vi "FSRCalibrationDataCollection.vi"() -> ()   [LabVIEW 2020]
doc: "Use this template to build a producer/consumer design pattern. Use this template when you need to execute a process, such as data analysis, when a data source, such as a triggered acquisition, produces data at an uneven rate and you need to execute the process when the data becomes available.\n------------------------------------\nAuther: Koji Ohashi\nCopyright (c) 2020 Japan LabVIEW Users Group, Volunteer members.\nThis VI is released under the MIT License.\nhttp://opensource.org/licenses/mit-license.php\n------------------------------------"
uses:
  FSRCalibrationDataCollection Folder/For fsr type def.ctl
  <vilib>/Analysis/baseanly.llb/Mean (DBL).vi
  <vilib>/Instr/_visa.llb/VISA Configure Serial Port (Instr).vi
  <vilib>/Analysis/NI_AALBase.lvlib
panel:
  out "Vout F4":dbl(slide) scale=0.0..2000.0
  out "Collecting":bool
  in  "Timer [ms]":u32
  out "On Time [ms]":u32
  out "millisecond timer":u32
  in  "Weight":T1(ring)
  out "Vout F1":dbl(slide) scale=0.0..2000.0
  in  "?":bool
  in  "Weight":string
  in  "Path":path=path "C:/Users/rsKite/Documents/FSR DATA"
  in  "Trial":string caption="Participant Name (FirstLast)"
  out "File Name":string
  out "Vout F3":dbl(slide) scale=0.0..2000.0
  out "Vout F2":dbl(slide) scale=0.0..2000.0
  out "Status":string
  in  "?":bool
  in  "VISA resource name":refnum<visa-resource-name>="COM1"
  in  "stop":bool
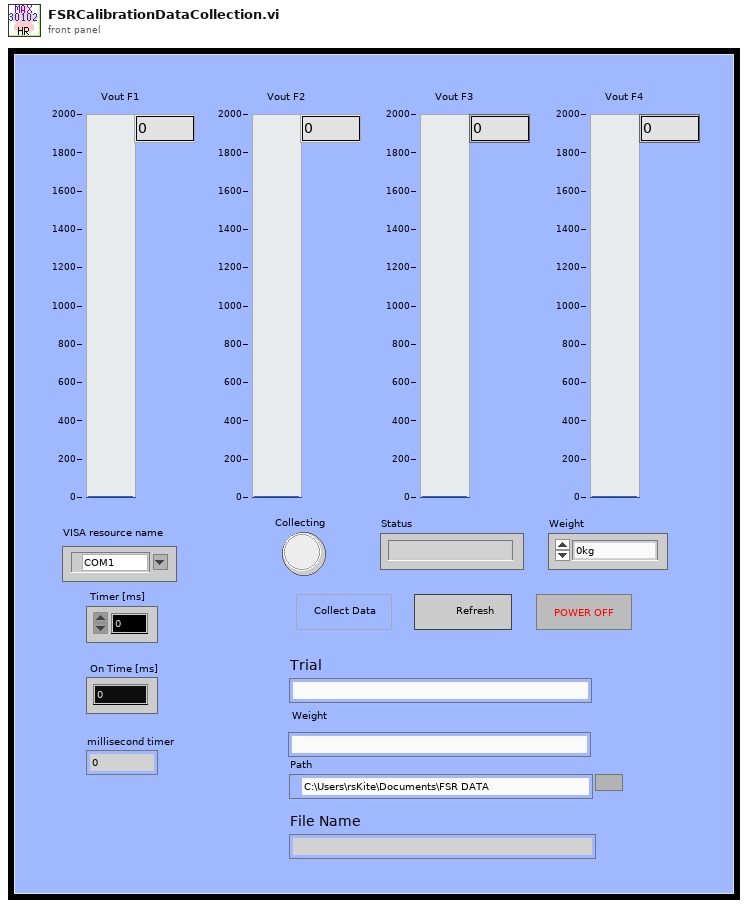
[diagram p1: front panel]
types:
  T1 = enum16{"0kg", "0.1kg", "0.2kg", "0.3kg", "0.4kg", "0.5kg", "0.6kg", "0.7kg", "0.8kg", "0.9kg", "1kg", "1.1kg", "1.2kg", "1.3kg", "1.4kg", "1.5kg", "1.6kg", "1.7kg", "1.8kg", "1.9kg", "2.0kg"}
  T2 = enum16{"open", "replace", "create", "open or create", "replace or create", "replace or create with confirmation"}
  T3 = typedef "For fsr type def.ctl" = enum16{"Create/Replace File", "Waiting Room", "Collect Data", "Write Data", "Close File", "Reinit"}
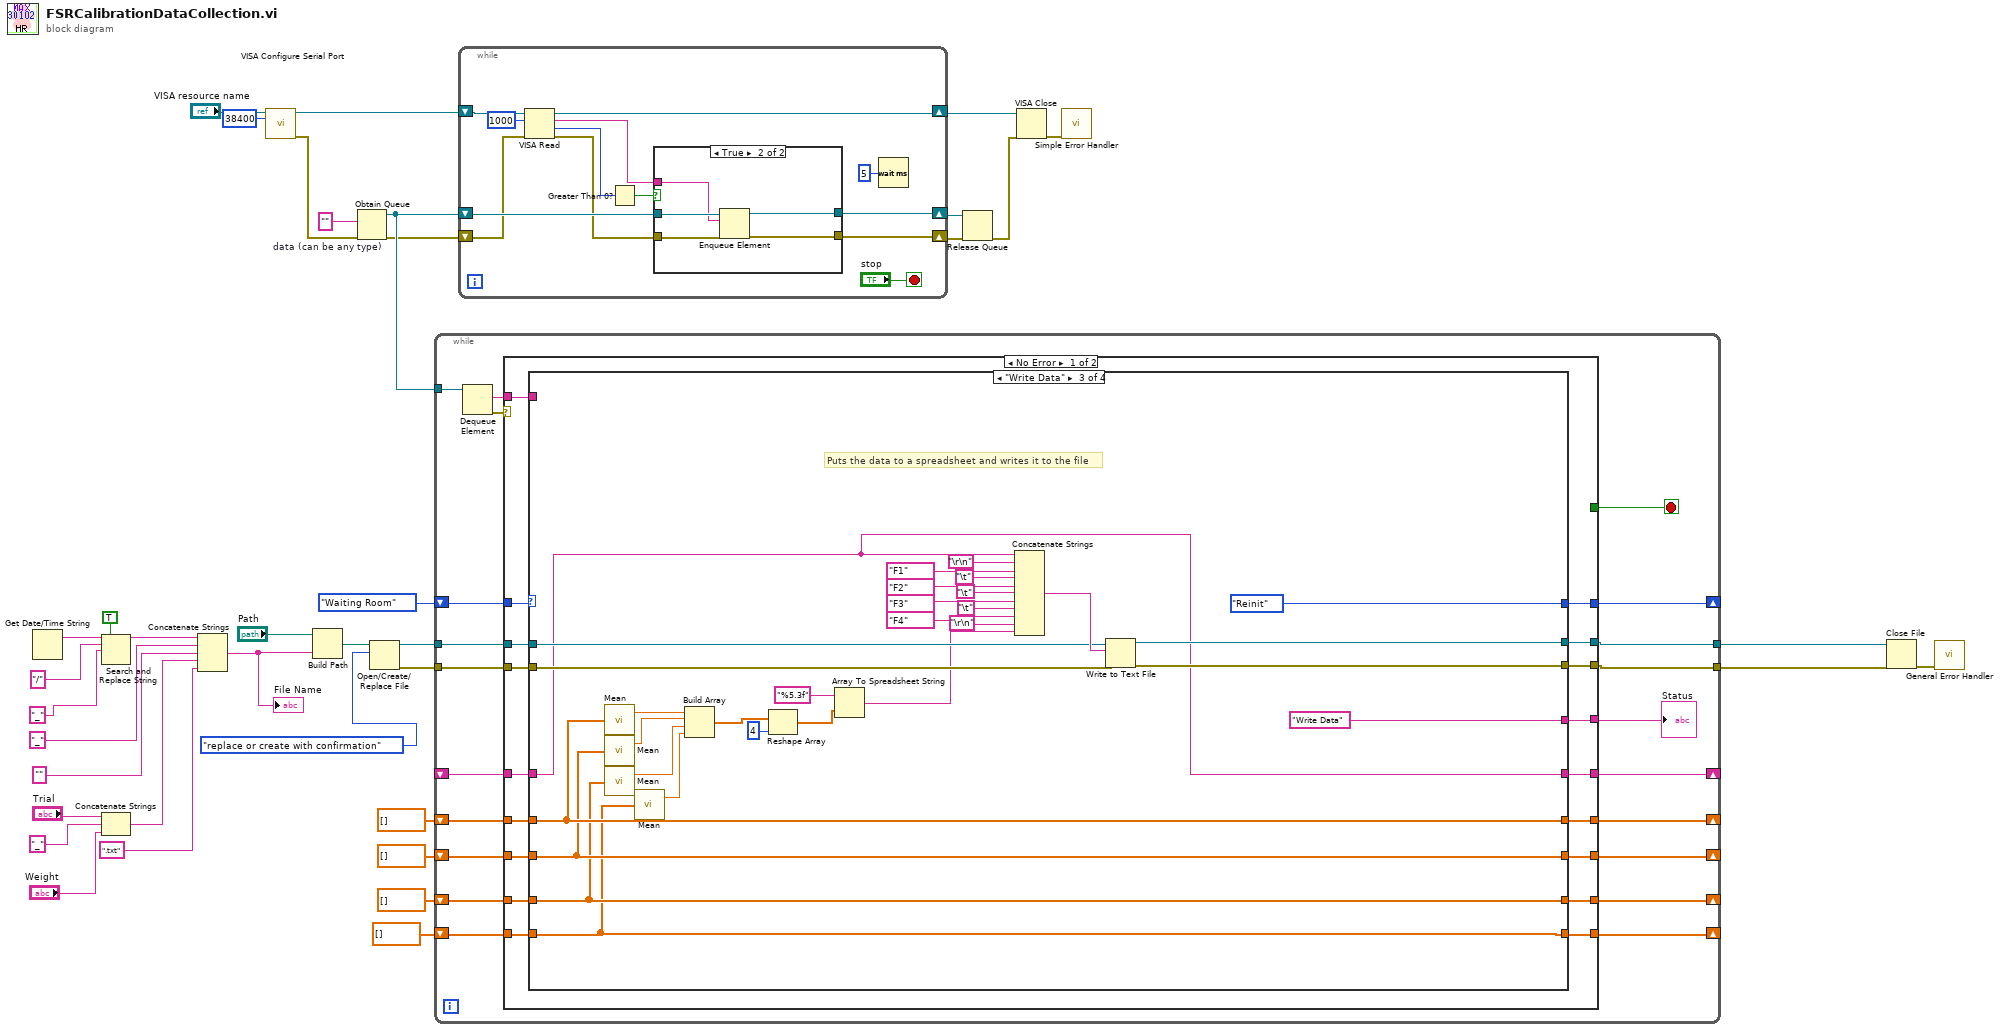
[diagram p0: block diagram]
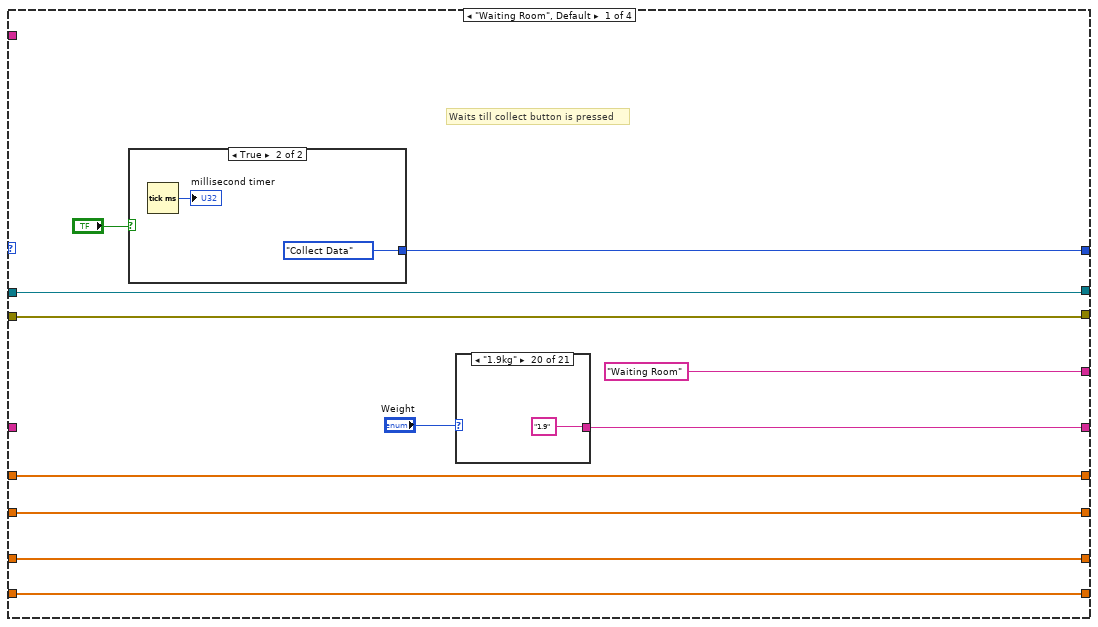
[diagram p2: hidden frame]
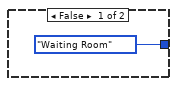
[diagram p3: hidden frame]
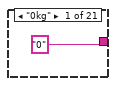
[diagram p4: hidden frame]
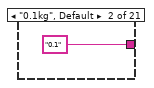
[diagram p5: hidden frame]
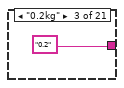
[diagram p6: hidden frame]
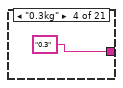
[diagram p7: hidden frame]
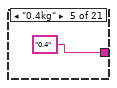
[diagram p8: hidden frame]
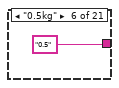
[diagram p9: hidden frame]
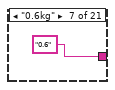
[diagram p10: hidden frame]
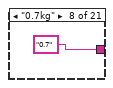
[diagram p11: hidden frame]
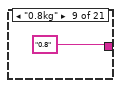
[diagram p12: hidden frame]
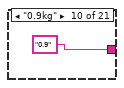
[diagram p13: hidden frame]
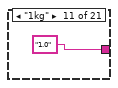
[diagram p14: hidden frame]
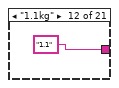
[diagram p15: hidden frame]
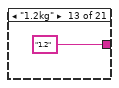
[diagram p16: hidden frame]
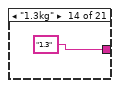
[diagram p17: hidden frame]
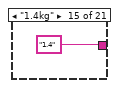
[diagram p18: hidden frame]
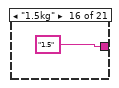
[diagram p19: hidden frame]
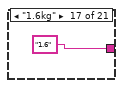
[diagram p20: hidden frame]
diagram:
  w34 = ""  # data (can be any type)
  n1 = Get Date/Time String() -> (date string=w25:string)  [unwired: 3 in, 1 out]
  n2 = Search and Replace String(replace all?=TRUE ("replace all? (F)"), input string=w25, search string="/", replace string="_" ("replace string (\"\")")) -> (result string=w23:string)  [unwired: 4 in, 3 out]
  n3 = Concatenate Strings("Trial", "_" ("string"), "Weight") -> (w24:string)
  n4 = Concatenate Strings(w23, "_" ("string"), "" ("string"), w24, ".txt" ("string")) -> (w21:string)
  "File Name" <- w21
  n5 = call-poly "VISA Configure Serial Port"("VISA resource name"="VISA resource name", "baud rate (9600)"=u32 38400) -> ("VISA resource name out"=w32:refnum<visa-resource-name>, "error out"=w29:errorcluster)  [unwired: 8 in, 4 out]
  n6 = Build Path(base path="Path", name or relative path=w21) -> (appended path=w10:path)
  n7 = Obtain Queue(element data type=w34, error in (no error)=w29) -> (queue out=w38:refnum<queue>, error out=w37:errorcluster)  [unwired: 3 in, 1 out]
  n8 = Open/Create/Replace File(file path (use dialog)=w10, operation (0:open)=T2."replace or create with confirmation") -> (refnum out=w8:refnum<file>, error out=w7:errorcluster)  [unwired: 4 in, 1 out]
  n9 = while {
    tunnel: w38 -> [w59]
    shift-right: [w53] -> _
    shift-left: For_fsr_type_def."Waiting Room" -> [w54]
    tunnel: w8 -> [w52]
    tunnel: w7 -> [w51]
    tunnel: [w50] -> w6
    tunnel: [w49] -> w5
    shift-right: [w45] -> _
    shift-left: dbl[] [] -> [w46]
    shift-right: [w47] -> _
    shift-left: dbl[] [] -> [w48]
    shift-right: [w43] -> _
    shift-left: dbl[] [] -> [w44]
    shift-right: [w41] -> _
    shift-left: _ -> [w42]
    shift-right: [w39] -> _
    shift-left: dbl[] [] -> [w40]
    stop <- w56 stop-if-true
    n10 = Dequeue Element(queue=w59) -> (element=w57:string, error out=w58:errorcluster)  [unwired: 2 in, 2 out]
    n11 = case shown="No Error" w58 {
      tunnel: w57 -> [w75 _]
      tunnel: [_ TRUE] -> w56
      tunnel: [w74 "Error or POWER OFF"] -> w55
      tunnel: w54 -> [w77 _]
      tunnel: [w76 For_fsr_type_def."Waiting Room"] -> w53
      tunnel: w52 -> [w73 w211]
      tunnel: w51 -> [w72 w210]
      tunnel: [w71 w211] -> w50
      tunnel: [w70 w210] -> w49
      tunnel: w48 -> [w69 w207]
      tunnel: [w68 w207] -> w47
      tunnel: w46 -> [w67 w208]
      tunnel: [w66 w208] -> w45
      tunnel: w44 -> [w65 w209]
      tunnel: [w64 w209] -> w43
      tunnel: w42 -> [w63 w206]
      tunnel: [w62 w206] -> w41
      tunnel: w40 -> [w61 w205]
      tunnel: [w60 w205] -> w39
      frame No Error {
        n12 = case shown="\"Write Data\"" w77 {
          tunnel: [w80 w122 For_fsr_type_def."Reinit" w189] -> w76
          tunnel: w75 -> [_ w142 _ _]
          tunnel: ["Waiting Room" "Collect data" "Write Data" "Reinit"] -> w74
          tunnel: w73 -> [w87 w140 w169 w191]
          tunnel: w72 -> [w86 w139 w168 w190]
          tunnel: [w87 w140 w167 w191] -> w71
          tunnel: [w86 w139 w166 w190] -> w70
          tunnel: w69 -> [w83 w136 w162 w183]
          tunnel: [w83 w118 w162 w186] -> w68
          tunnel: w67 -> [w84 w133 w163 w184]
          tunnel: [w84 w131 w163 w187] -> w66
          tunnel: w65 -> [w85 w132 w164 w185]
          tunnel: [w85 w130 w164 w188] -> w64
          tunnel: [w82 w128 w154 w180] -> w62
          tunnel: w63 -> [_ w128 w154 w181]
          tunnel: w61 -> [w78 w116 w153 w179]
          tunnel: [w78 w115 w153 w178] -> w60
          frame "Waiting Room", Default {
            # "Waits till collect button is pressed"
            n13 = case shown="True" "?" {
              tunnel: [For_fsr_type_def."Waiting Room" For_fsr_type_def."Collect Data"] -> w80
              frame False {
              }
              frame True {
                n14 = Tick Count (ms)() -> (millisecond timer value=→"millisecond timer":u32)
              }
            }
            n15 = case shown="\"1.9kg\"" "Weight" {
              tunnel: ["0" "0.1" "0.2" "0.3" "0.4" "0.5" "0.6" "0.7" "0.8" "0.9" "1.0" "1.1" "1.2" "1.3" "1.4" "1.5" "1.6" "1.7" "1.8" "1.9" "2.0"] -> w82
              frame "0kg" {
              }
              frame "0.1kg", Default {
              }
              frame "0.2kg" {
              }
              frame "0.3kg" {
              }
              frame "0.4kg" {
              }
              frame "0.5kg" {
              }
              frame "0.6kg" {
              }
              frame "0.7kg" {
              }
              frame "0.8kg" {
              }
              frame "0.9kg" {
              }
              frame "1kg" {
              }
              frame "1.1kg" {
              }
              frame "1.2kg" {
              }
              frame "1.3kg" {
              }
              frame "1.4kg" {
              }
              frame "1.5kg" {
              }
              frame "1.6kg" {
              }
              frame "1.7kg" {
              }
              frame "1.8kg" {
              }
              frame "1.9kg" {
              }
              frame "2.0kg" {
              }
            }
          }
          frame "Collect Data" {
            w119 = ","
            # "Collects data from Arduino\n Stops when timer is up"
            n16 = Match Pattern(string=w142, regular expression=w119) -> (before substring=w138:string, after substring=w137:string)  [unwired: 1 in, 2 out]
            n17 = Match Pattern(string=w137, regular expression=w119) -> (before substring=w141:string, after substring=w114:string)  [unwired: 1 in, 2 out]
            n18 = Fract/Exp String To Number(string=w138) -> (number=w129:dbl)  [unwired: 3 in, 1 out]
            "Vout F1" <- w129
            n19 = Match Pattern(string=w114, regular expression=w119) -> (before substring=w113:string, after substring=w120:string)  [unwired: 1 in, 2 out]
            n20 = Fract/Exp String To Number(string=w141) -> (number=w134:dbl)  [unwired: 3 in, 1 out]
            "Vout F2" <- w134
            n21 = Fract/Exp String To Number(string=w120) -> (number=w117:dbl)  [unwired: 3 in, 1 out]
            "Vout F4" <- w117
            n22 = Fract/Exp String To Number(string=w113) -> (number=w135:dbl)  [unwired: 3 in, 1 out]
            "Vout F3" <- w135
            n23 = Build Array (concatenate)(w132, w129) -> (w130:dbl[])
            n24 = Build Array (concatenate)(w136, w135) -> (w118:dbl[])
            n25 = Build Array (concatenate)(w133, w134) -> (w131:dbl[])
            n26 = Build Array (concatenate)(w116, w117) -> (w115:dbl[])
            n27 = local read "millisecond timer"() -> (w124:u32)
            n28 = Tick Count (ms)() -> (millisecond timer value=w127:u32)
            n29 = Subtract(x=w127, y=w124) -> (x-y=w126:u32)
            "On Time [ms]" <- w126
            n30 = Greater?(x=w126, y="Timer [ms]") -> (0:w121:bool)
            n31 = case shown="False" w121 {
              tunnel: [TRUE FALSE] -> w123
              tunnel: [For_fsr_type_def."Collect Data" For_fsr_type_def."Write Data"] -> w122
              frame False {
              }
              frame True {
              }
            }
            "Collecting" <- w123
          }
          frame "Write Data" {
            # "Puts the data to a spreadsheet and writes it to the file"
            n32 = call-poly <vilib>:"Mean.vi"("X"=w164) -> ("mean"=w161:dbl)  [unwired: 1 out]
            n33 = call-poly <vilib>:"Mean.vi"("X"=w163) -> ("mean"=w160:dbl)  [unwired: 1 out]
            n34 = call-poly <vilib>:"Mean.vi"("X"=w162) -> ("mean"=w159:dbl)  [unwired: 1 out]
            n35 = call-poly <vilib>:"Mean.vi"("X"=w153) -> ("mean"=w152:dbl)  [unwired: 1 out]
            n36 = Build Array(w161, w160, w159, w152) -> (w157:dbl[])
            n37 = Reshape Array(w157, 4 ("dimension size")) -> (w158:dbl[])
            n38 = Array To Spreadsheet String(array=w158, 3:"%5.3f" ("format string")) -> (spreadsheet string=w148:string)  [unwired: 1 in]
            n39 = Concatenate Strings(w154, "\r\n", "F1", "\t", "F2", "\t", "F3", "\t", "F4", "\r\n", w148) -> (w174:string)
            n40 = Write to Text File(file (use dialog)=w169, text=w174, error in=w168) -> (refnum out=w167:refnum<file>, error out=w166:errorcluster)  [unwired: 1 in, 1 out]
          }
          frame "Reinit" {
            # "Clears data previously collected"
            n41 = case shown="False" "?" {
              tunnel: [For_fsr_type_def."Reinit" For_fsr_type_def."Waiting Room"] -> w189
              tunnel: [w198 dbl[] []] -> w188
              tunnel: [w197 dbl[] []] -> w187
              tunnel: [w196 dbl[] []] -> w186
              tunnel: w185 -> [w198 _]
              tunnel: w184 -> [w197 _]
              tunnel: w183 -> [w196 _]
              tunnel: w181 -> [w194 _]
              tunnel: [w194 ""] -> w180
              tunnel: w179 -> [w193 _]
              tunnel: [w193 dbl[] []] -> w178
              frame False {
              }
              frame True {
              }
            }
          }
        }
      }
      frame Error {
      }
    }
    "Status" <- w55
  }
  n42 = while {
    shift-right: [w224] -> w35
    shift-left: w37 -> [w218]
    shift-right: [w225] -> w36
    shift-left: w38 -> [w226]
    shift-right: [w222] -> w30
    shift-left: w32 -> [w216]
    stop <- "stop" stop-if-true
    n43 = VISA Read(VISA resource name=w216, byte count=u32 1000, error in (no error)=w218) -> (VISA resource name out=w222:refnum<visa-resource-name>, read buffer=w219:string, return count=w221:u32, error out=w217:errorcluster)
    n44 = Greater Than 0?(x=w221) -> (x > 0?=w220:bool)
    n45 = case shown="True" w220 {
      tunnel: w226 -> [w229 w234]
      tunnel: [w229 w233] -> w225
      tunnel: w217 -> [w228 w232]
      tunnel: [w228 w231] -> w224
      tunnel: w219 -> [_ w230]
      frame False {
      }
      frame True {
        n46 = Enqueue Element(queue=w234, element=w230, error in (no error)=w232) -> (queue out=w233:refnum<queue>, error out=w231:errorcluster)  [unwired: 1 in, 1 out]
      }
    }
    n47 = Wait (ms)(milliseconds to wait=u32 5) -> ()  [unwired: 1 out]
  }
  n48 = Release Queue(queue=w36, error in (no error)=w35) -> (error out=w28:errorcluster)  [unwired: 1 in, 2 out]
  n49 = VISA Close(VISA resource name=w30, error in (no error)=w28) -> (error out=w31:errorcluster)
  n50 = call <vilib>:"Simple Error Handler.vi"("error in (no error)"=w31) -> ()  [unwired: 1 in, 8 out]
  n51 = Close File(refnum=w6, error in=w5) -> (error out=w9:errorcluster)  [unwired: 1 out]
  n52 = call <vilib>:"General Error Handler.vi"("error in (no error)"=w9) -> ()  [unwired: 10 in, 5 out]
